vi "identification.vi"(2 "Password":string, 3 "Identifiant":string) -> (0 "role":string, 1 "prenom":string)   [LabVIEW 2024]
uses:
  <vilib>/drjdpowell/SQLite Library/SQL Connection/Open (string).vi
  <vilib>/drjdpowell/SQLite Library/SQL Connection/Execute SQL.vi
  <vilib>/drjdpowell/SQLite Library/SQL Connection/Connection.lvclass
  <vilib>/drjdpowell/SQLite Library/SQLite.lvlib
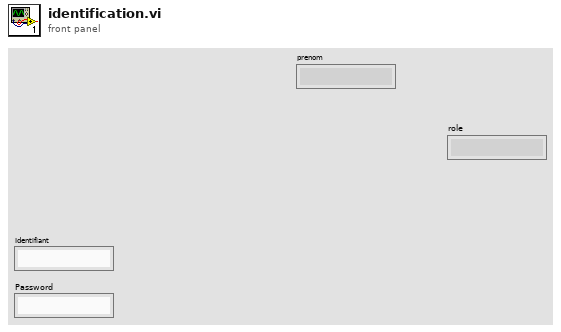
[diagram p1: front panel]
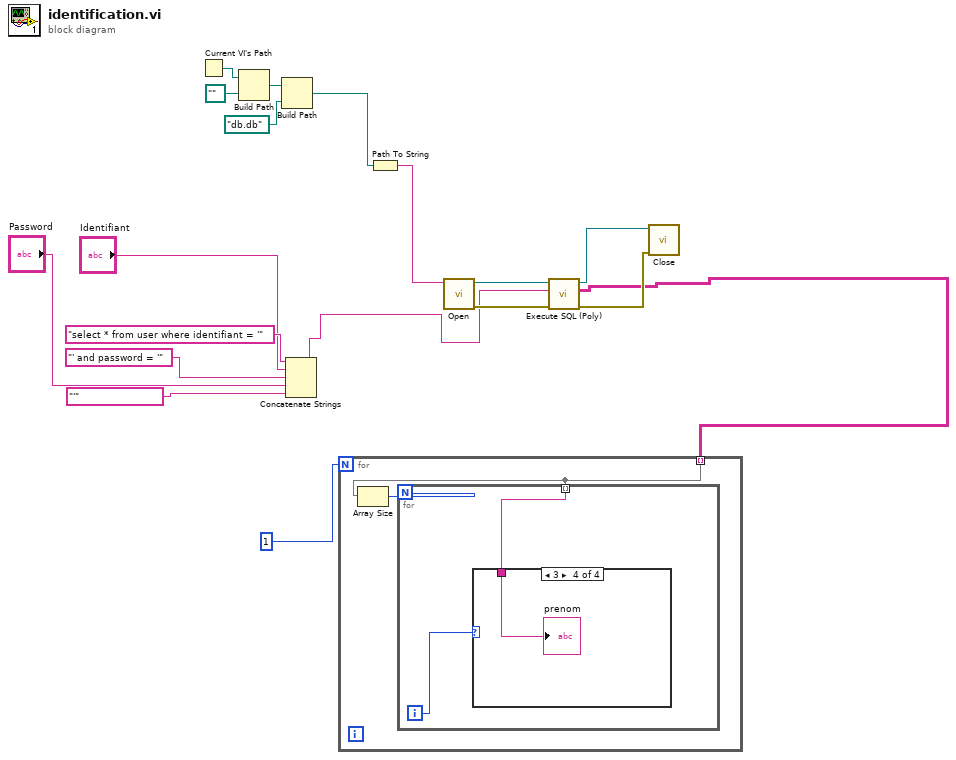
[diagram p0: block diagram]
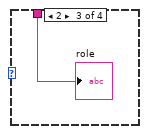
[diagram p4: hidden frame]
diagram:
  n1 = Current VI's Path() -> (path=w6:path)
  n2 = Build Path(base path=w6, name or relative path=path "..") -> (appended path=w3:path)
  n3 = Build Path(base path=w3, name or relative path=path "db.db" ("Filename")) -> (appended path=w2:path)
  n4 = Concatenate Strings("select * from user where identifiant = '", "Identifiant", "' and password = '", "Password", "'") -> (w8:string)
  n5 = Path To String(path=w2) -> (string=w1:string)
  n6 = call-poly <vilib>:"Open.vi"("db file"=w1) -> ("error out"=w11:errorcluster, "SQLite Connection"=w12:refnum<class "Connection.lvclass">)  [unwired: 9 in]
  n7 = call-poly <vilib>:"Execute SQL (Poly).vi"("error in (no error)"=w11, "SQL"=w8, "SQLite Connection in"=w12) -> ("error out"=w10:errorcluster, "Result Set"=w7:string[][], "SQLite Connection"=w9:refnum<class "Connection.lvclass">)  [unwired: 5 in, 1 out]
  n8 = for {
    N: 1 -> [_]
    tunnel: w7 -> [w19] mode=indexing
    n9 = Array Size(array=w19) -> (size(s)=w20:i32)
    n10 = for {
      N: w20 -> [_]
      tunnel: w19 -> [w21] mode=indexing
      i -> [w22]
      n11 = case shown="3" w22 {
        tunnel: w21 -> [_ _ w23 w24]
        frame 0, Default {
        }
        frame 1 {
        }
        frame 2 {
          "role" <- w23
        }
        frame 3 {
          "prenom" <- w24
        }
      }
    }
  }
  n12 = call-dynamic "Close.vi"("error in (no error)"=w10, "SQLite Connection in"=w9) -> ()  [unwired: 9 in, 1 out]
